vi "util_set_change_in.vi"(7 "references":T1, 8 "error in (no error)":errorcluster, 10 "data":variant, 11 "change":bool) -> (0 "error out":errorcluster)   [LabVIEW 2015, in "repub-dvr_nre.lvlib"]
uses:
  repub-dvr_nre.lvlib
  _controls/references.ctl
  private/_controls/input.ctl
  private/_controls/input_command.ctl
  private/_controls/output.ctl
  private/_controls/data.ctl
  _controls/configuration.ctl
  lv-recipe-machine/private/_controls/recipe_data.ctl
  lv-recipe-machine/public/_controls/mode.ctl
  lv-recipe-machine/public/_controls/manual_state.ctl
  lv-recipe-machine/public/_controls/automatic_state.ctl
  <userlib>/antonio-alexander/lv-waitgroup/public/_controls/api_waitgroup.ctl
  lv-recipe-machine/public/_controls/transition.ctl
  _controls/change.ctl
  _controls/status.ctl
  lv-recipe-machine/lv-recipe-machine.lvlib
  <userlib>/antonio-alexander/lv-waitgroup/lv-waitgroup.lvlib
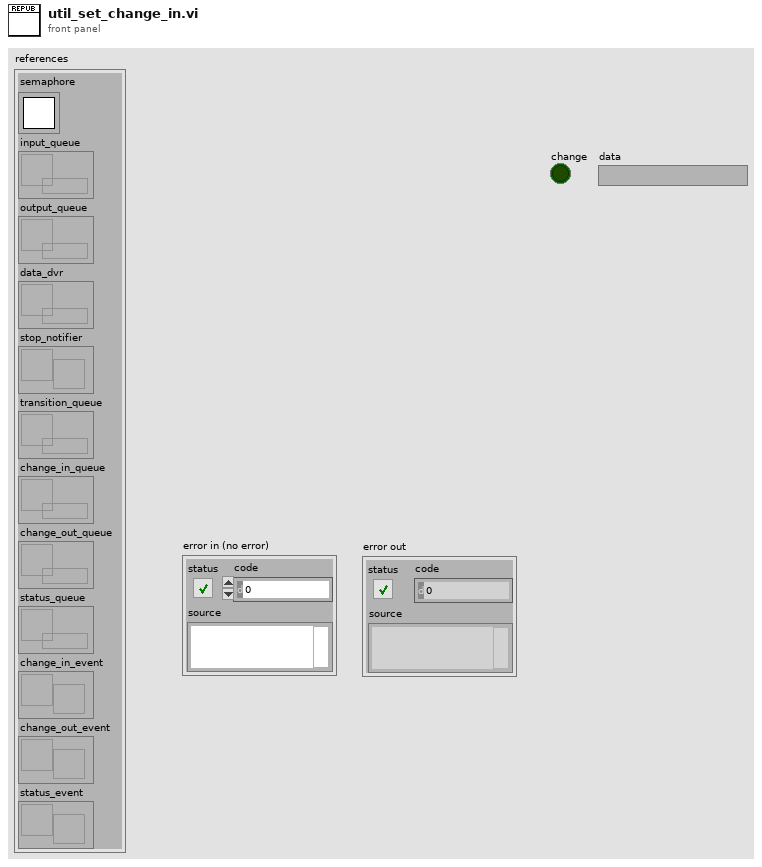
[diagram p1: front panel]
types:
  T1 = typedef "repub-dvr_nre.lvlib/references.ctl" = cluster{"semaphore":T2, "input_queue":refnum<queue>, "output_queue":refnum<queue>, "data_dvr":refnum<data-value>, "stop_notifier":refnum<notifier>, "transition_queue":refnum<queue>, "change_in_queue":refnum<queue>, "change_out_queue":refnum<queue>, "status_queue":refnum<queue>, "change_in_event":refnum<user-event>, "change_out_event":refnum<user-event>, "status_event":refnum<user-event>}
  T2 = typedef "Semaphore RefNum" = refnum<k1>
  T3 = typedef "repub-dvr_nre.lvlib/change.ctl" = cluster{"changed":bool, "data":variant}
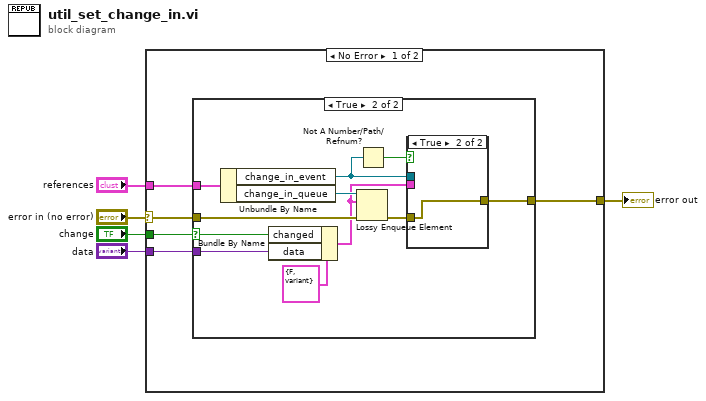
[diagram p0: block diagram]
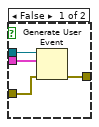
[diagram p3: hidden frame]
diagram:
  n1 = case shown="No Error" "error in (no error)" {
    selector: "error in (no error)" -> [w9 w28]
    tunnel: [w6 w28] -> w4
    tunnel: "references" -> [w10 _]
    tunnel: "change" -> [w8 _]
    tunnel: "data" -> [w7 _]
    frame No Error {
      n2 = case shown="True" w8 {
        selector: w8 -> [_ w18]
        tunnel: w10 -> [_ w22]
        tunnel: w9 -> [w11 w20]
        tunnel: w7 -> [_ w17]
        tunnel: [w11 w14] -> w6
        frame False {
        }
        frame True {
          n3 = Unbundle By Name(w22) -> ("change_in_event"=w13:refnum<user-event>, "change_in_queue"=w21:refnum<queue>)
          n4 = Bundle By Name(cluster=T3 {"changed"=FALSE, "data"=variant} ("change"), "changed"=w18, "data"=w17) -> (w16:T3)
          n5 = Lossy Enqueue Element(queue=w21, element=w16, error in (no error)=w20) -> (error out=w15:errorcluster)  [unwired: 3 out]
          n6 = Not A Number/Path/Refnum?(number/path/refnum=w13) -> (NaN/Path/Refnum?=w12:bool)
          n7 = case shown="True" w12 {
            tunnel: w16 -> [w26 _]
            tunnel: w15 -> [w25 w27]
            tunnel: [w24 w27] -> w14
            tunnel: w13 -> [w23 _]
            frame False {
              n8 = Generate User Event(user event=w23, event data cluster=w26, error in=w25) -> (error out=w24:errorcluster)  [unwired: 1 in, 1 out]
            }
            frame True {
            }
          }
        }
      }
    }
    frame Error {
    }
  }
  "error out" <- w4
